vi "bin.vi"() -> ()   [LabVIEW 2013]
panel:
  in  "data #":i32
  out "taustream":dbl[][](array[numeric])
  out "matlab error":errorcluster
  out "data":dbl[](array[numeric]) format="%#.6f"
  in  "extra":dbl
  in  "yPixels":dbl
  in  "xPixels":dbl
  in  "sAOxy":dbl
  in  "sample rate":dbl
  in  "frame time":dbl
  in  "resolution":dbl
  in  "sync time":dbl
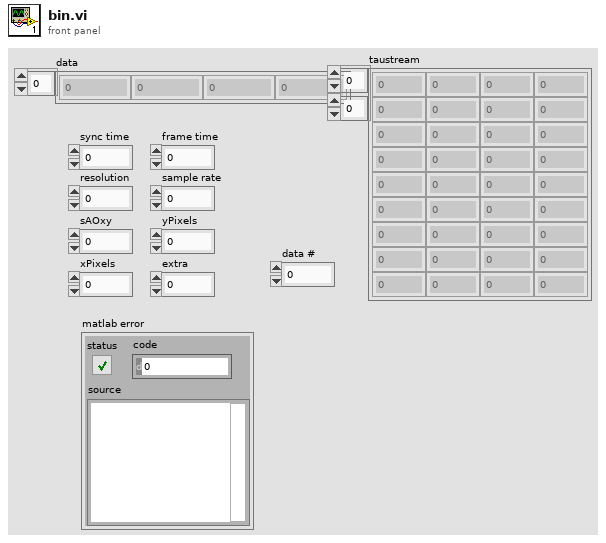
[diagram p1: front panel]
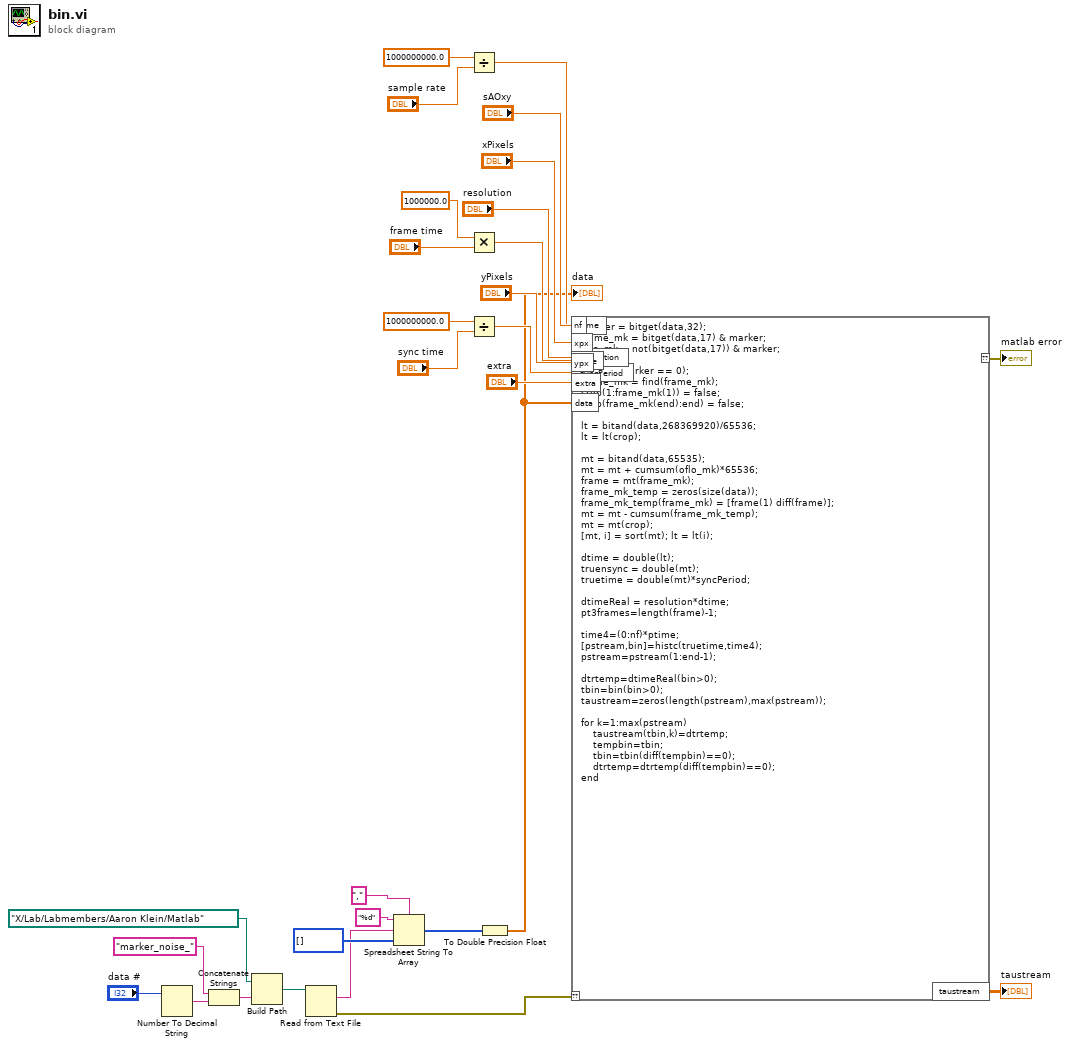
[diagram p0: block diagram]
diagram:
  n1 = Number To Decimal String(number="data #") -> (decimal integer string=w8:string)  [unwired: 1 in]
  n2 = Concatenate Strings("marker_noise_" ("string"), w8) -> (w12:string)
  n3 = Build Path(base path=path "X:/Lab/Labmembers/Aaron Klein/Matlab", name or relative path=w12) -> (appended path=w11:path)
  n4 = Read from Text File(file (use dialog)=w11) -> (text=w4:string, error out=w1:errorcluster)  [unwired: 3 in, 2 out]
  n5 = Spreadsheet String To Array(delimiter (Tab)=",", format string="%d", spreadsheet string=w4, array type (2D Dbl)=i64[] []) -> (array=w3:i64[])
  n6 = Divide(x=1000000000.0, y="sample rate") -> (x/y=w16:dbl)
  n7 = Multiply(x=1000000.0, y="frame time") -> (x*y=w20:dbl)
  n8 = Divide(x=1000000000.0, y="sync time") -> (x/y=w22:dbl)
  n9 = To Double Precision Float(number=w3) -> (double precision float=w2:dbl[])
  "data" <- w2
  n10 = script code="marker = bitget(data,32);\nframe_mk = bitget(data,17) & marker;\noflo_mk = not(bitget(data,17)) & marker;\n\ncrop = (marker == 0);\nframe_mk = find(frame_mk);\ncrop(1:frame_mk(1)) = false;\ncrop(frame_mk(end):end) = false;\n\nlt = bitand(data,268369920)/65536;\nlt = lt(crop);\n\nmt = bitand(data,65535);\nmt = mt + cumsum(oflo_mk)*65536;\nframe = mt(frame_mk);\nframe_mk_temp = zeros(size(data));\nframe_mk_temp(frame_mk) = [frame(1) diff(frame)];\nmt = mt - cumsum(frame_mk_temp);\nmt = mt(crop);\n[mt, i] = sort(mt); lt = lt(i);\n\ndtime = double(lt);\ntruensync = double(mt);\ntruetime = double(mt)*syncPeriod;\n\ndtimeReal = resolution*dtime;\npt3frames=length(frame)-1;\n\ntime4=(0:nf)*ptime;\n[pstream,bin]=histc(truetime,time4);\npstream=pstream(1:end-1);\n\ndtrtemp=dtimeReal(bin>0);\ntbin=bin(bin>0);\ntaustream=zeros(length(pstream),max(pstream));\n\nfor k=1:max(pstream)\n    taustream(tbin,k)=dtrtemp;\n    tempbin=tbin;\n    tbin=tbin(diff(tempbin)==0);\n    dtrtemp=dtrtemp(diff(tempbin)==0);\nend"("??"=w1, "syncPeriod"=w22, "resolution"="resolution", "ftime"=w20, "ptime"=w16, "nf"="sAOxy", "xpx"="xPixels", "ypx"="yPixels", "extra"="extra", "data"=w2) -> ("??"=→"matlab error":errorcluster, "taustream"=→"taustream":dbl[][])
